vi "w_r_bin.vi"() -> ()   [LabVIEW 2020]
uses:
  <vilib>/Utility/file.llb/Read Delimited Spreadsheet (string).vi
panel:
  out "length 2":i32
  out "length":i32
  out "Array 3":i32[](array[numeric])
  out "String":string
  out "size(s)":i32
  out "Numeric":i32
  out "w_bin_data":string
  out "polarity":string
  out "mode":string
  out "error out":errorcluster
  in  "binFile_bin":path=path "D:/_Project/_Code/LabVIEW/CLC_Gen4/L2_Cali/CLC_Gen4_L2_InPhaseCal_Power/Config/bin/VinceTest.bin"
  out "Array 2":string[](array[string])
  out "Array":i32[][](array[numeric])
  out "all rows":string[][](array[string])
  in  "InPhase_Table_CSV":path=path "D:/_Project/_Code/LabVIEW/CLC_Gen4/L2_Cali/CLC_Gen4_L2_InPhaseCal_Power/Config/In-Phase_setting/In_phase_Table_20240904_134023_43.csv"
  out "r_bin_data":string
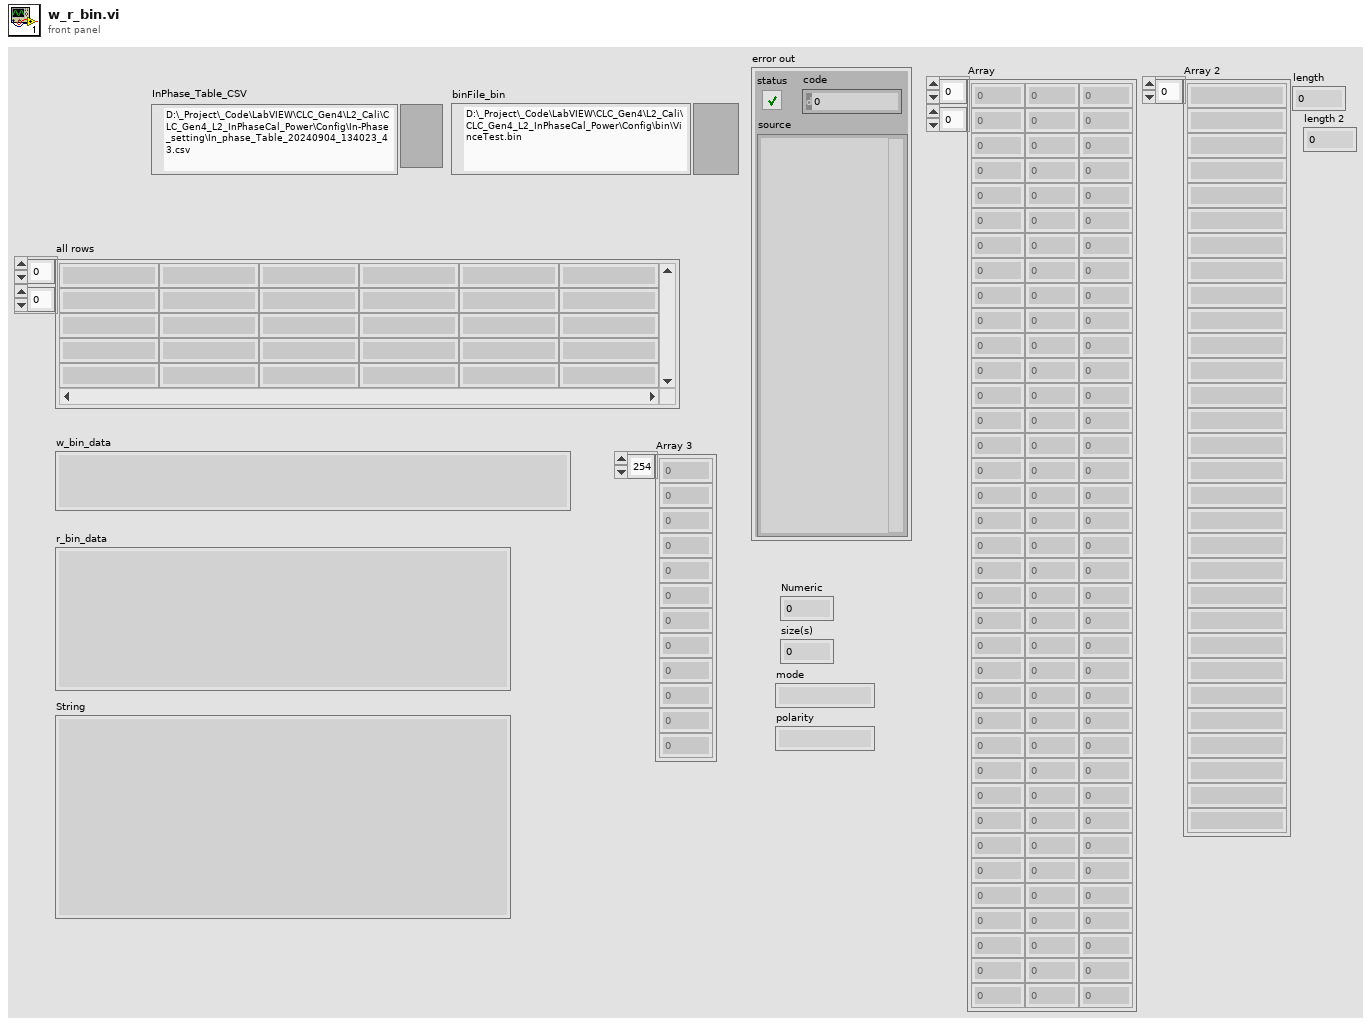
[diagram p1: front panel]
types:
  T1 = enum16{"open", "replace", "create", "open or create", "replace or create", "replace or create with confirmation"}
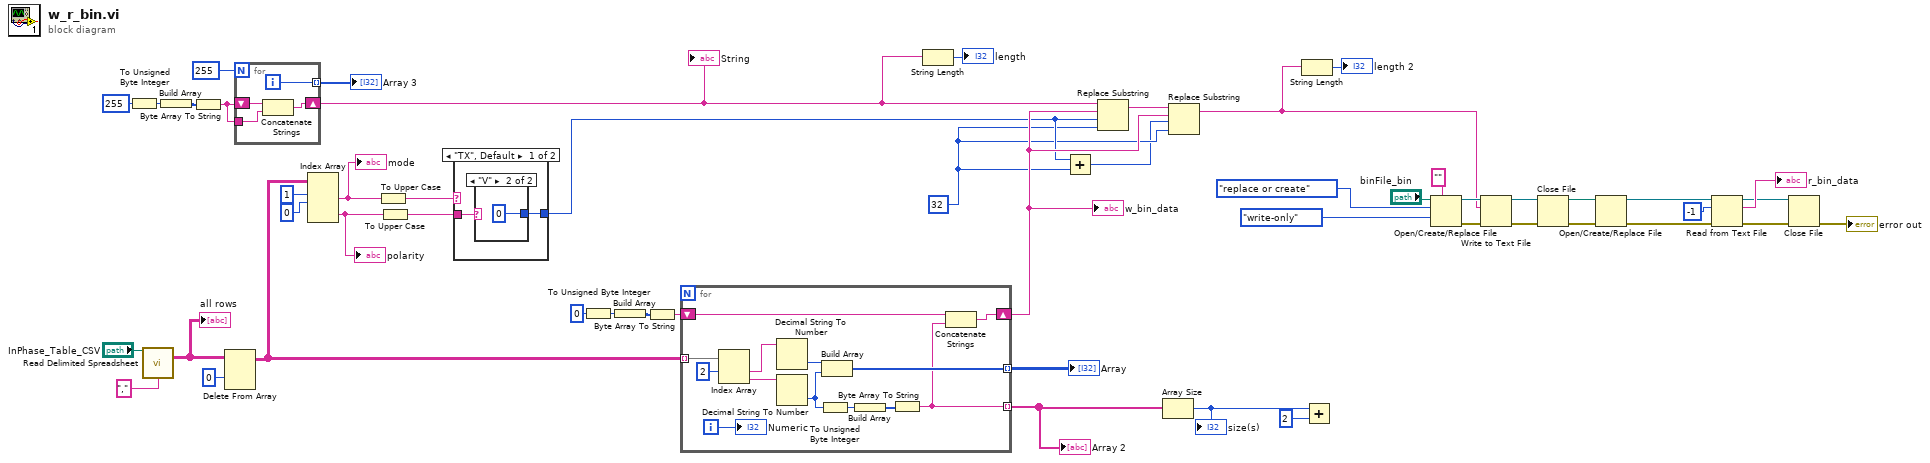
[diagram p0: block diagram]
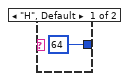
[diagram p2: hidden frame]
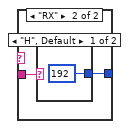
[diagram p3: hidden frame]
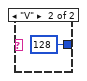
[diagram p4: hidden frame]
diagram:
  w11 = 32 ("length (len. of substring)")
  n1 = To Unsigned Byte Integer(number=u8 255) -> (unsigned 8bit integer=w8:u8)
  n2 = call-poly <vilib>:"Read Delimited Spreadsheet.vi"("file path (dialog if empty)"="InPhase_Table_CSV", "delimiter (\\t)"="," ("delimiter (\\t)")) -> ("all rows"=w49:string[][])  [unwired: 8 in, 5 out]
  "all rows" <- w49
  n3 = Build Array(w8) -> (w9:u8[])
  n4 = Byte Array To String(unsigned byte array=w9) -> (string=w6:string)
  n5 = Delete From Array(array=w49, index (row)=0) -> (array with subset deleted=w27:string[][])  [unwired: 2 in, 1 out]
  n6 = for {
    N: 255 -> [_]
    shift-right: [w55] -> w4
    shift-left: w6 -> [w54]
    tunnel: w6 -> [w53]
    tunnel: [w52] -> w5 mode=indexing
    i -> [w52]
    n7 = Concatenate Strings(w54, w53) -> (w55:string)
  }
  "String" <- w4
  "Array 3" <- w5
  n8 = Index Array(array=w27, index (row) #1=1 ("index (row)"), index (col) #1=0 ("disabled index (col)")) -> (element #1=w19:string, element #2=w18:string)  [unwired: 2 in]
  "mode" <- w19
  "polarity" <- w18
  n9 = To Upper Case(1:w19) -> (0:w17:string)
  n10 = To Upper Case(1:w18) -> (0:w16:string)
  n11 = case shown="\"TX\", Default" w17 {
    tunnel: w16 -> [w57 w61]
    tunnel: [w56 w60] -> w12
    frame "TX", Default {
      n12 = case shown="\"V\"" w57 {
        tunnel: [64 ("offset (0)") 0 ("offset (0)")] -> w56
        frame "H", Default {
        }
        frame "V" {
        }
      }
    }
    frame "RX" {
      n13 = case shown="\"H\", Default" w61 {
        tunnel: [192 ("offset (0)") 128 ("offset (0)")] -> w60
        frame "H", Default {
        }
        frame "V" {
        }
      }
    }
  }
  n14 = To Unsigned Byte Integer(number=u8 0) -> (unsigned 8bit integer=w43:u8)
  n15 = Build Array(w43) -> (w44:u8[])
  n16 = Byte Array To String(unsigned byte array=w44) -> (string=w41:string)
  n17 = for {
    tunnel: w27 -> [w71] mode=indexing
    tunnel: [w75] -> w47 mode=indexing
    tunnel: [w65] -> w45 mode=indexing
    shift-right: [w66] -> w13
    shift-left: w41 -> [w67]
    i -> [w64]
    n18 = Index Array(array=w71, index #1=2 ("index")) -> (element #1=w70:string, element #2=w68:string)  [unwired: 1 in]
    n19 = Decimal String To Number(string=w70) -> (number=w76:i32)  [unwired: 2 in, 1 out]
    n20 = Decimal String To Number(string=w68) -> (number=w74:i32)  [unwired: 2 in, 1 out]
    n21 = To Unsigned Byte Integer(number=w74) -> (unsigned 8bit integer=w73:u8)
    n22 = Build Array(w76, w74) -> (w75:i32[])
    n23 = Build Array(w73) -> (w72:u8[])
    n24 = Byte Array To String(unsigned byte array=w72) -> (string=w65:string)
    n25 = Concatenate Strings(w67, w65) -> (w66:string)
    "Numeric" <- w64
  }
  "Array" <- w47
  "Array 2" <- w45
  "w_bin_data" <- w13
  n26 = String Length(string=w4) -> (length=→"length":i32)
  n27 = Add(x=w12, y=w11) -> (x+y=w10:i32)
  n28 = Replace Substring(2:w11, 3:w12, 4:w13, 5:w4) -> (1:w14:string)  [unwired: 1 out]
  n29 = Array Size(array=w45) -> (size(s)=w22:i32)
  "size(s)" <- w22
  n30 = Replace Substring(2:w11, 3:w10, 4:w13, 5:w14) -> (1:w1:string)  [unwired: 1 out]
  n31 = String Length(string=w1) -> (length=→"length 2":i32)
  n32 = Add(x=w22, y=2) -> ()  [unwired: 1 out]
  n33 = Open/Create/Replace File(file path (use dialog)="binFile_bin", prompt="", operation (0:open)=T1."replace or create", access (0:read/write)=enum16{"read/write", "read-only", "write-only"}."write-only") -> (refnum out=w39:refnum<file>, error out=w40:errorcluster)  [unwired: 2 in, 1 out]
  n34 = Write to Text File(file (use dialog)=w39, text=w1, error in=w40) -> (refnum out=w36:refnum<file>, error out=w37:errorcluster)  [unwired: 1 in, 1 out]
  n35 = Close File(refnum=w36, error in=w37) -> (path=w34:path, error out=w35:errorcluster)
  n36 = Open/Create/Replace File(file path (use dialog)=w34, error in=w35) -> (refnum out=w23:refnum<file>, error out=w31:errorcluster)  [unwired: 4 in, 1 out]
  n37 = Read from Text File(file (use dialog)=w23, count=-1, error in=w31) -> (refnum out=w32:refnum<file>, text=→"r_bin_data":string, error out=w33:errorcluster)  [unwired: 1 in, 1 out]
  n38 = Close File(refnum=w32, error in=w33) -> (error out=→"error out":errorcluster)  [unwired: 1 out]
